vi "MU Get Config.vi"(8 "error in (no error)":errorcluster, 10 "configuration":u32, 11 "handle":u64) -> (0 "error out (no error)":errorcluster, 2 "value":u32, 3 "function return":u32)   [LabVIEW 2017, in "MU_3SL_interface.lvlib"]
uses:
  MU_3SL_interface.lvlib
  lib/MU_3SL_interface.dll
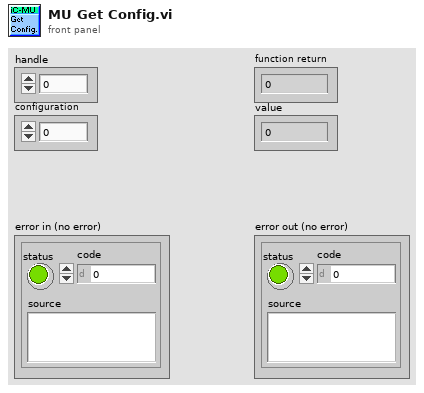
[diagram p1: front panel]
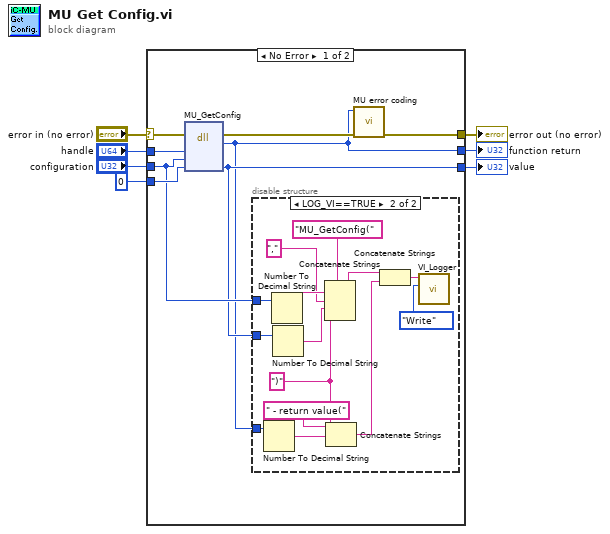
[diagram p0: block diagram]
diagram:
  n1 = case shown="No Error" "error in (no error)" {
    selector: "error in (no error)" -> [w13 w31]
    tunnel: [w8 w30] -> w7
    tunnel: "handle" -> [w11 _]
    tunnel: "configuration" -> [w10 _]
    tunnel: [w9 w30] -> w4
    tunnel: [w14 w31] -> w3
    tunnel: u32 0 ("pulValue") -> [w12 w30]
    frame No Error {
      n2 = dll-call lib="C:/Users/bes/AppData/Roaming/work/mu_9so/icsubmodules/soft_mu_3sl_master/lv_interface/lib/MU_3SL_interface**.*" fn="MU_GetConfig"(error in=w13, "handle"=w11, "configuration"=w10, "value"=w12) -> (error out=w15:errorcluster, "return type"=w8:u32, "value"=w9:u32)  [unwired: 4 in, 1 out]
      n3 = disable-structure shown="LOG_VI==TRUE" {
        disable-tunnel: w8 -> [_ w27]
        disable-tunnel: w10 -> [_ w22]
        disable-tunnel: w9 -> [_ w19]
        frame condition #0 {
        }
        frame condition #1 (active) {
          w16 = ")" ("string")
          n4 = Number To Decimal String(number=w27) -> (decimal integer string=w26:string)  [unwired: 1 in]
          n5 = Number To Decimal String(number=w22) -> (decimal integer string=w21:string)  [unwired: 1 in]
          n6 = Number To Decimal String(number=w19) -> (decimal integer string=w18:string)  [unwired: 1 in]
          n7 = Concatenate Strings("MU_GetConfig(" ("Info in"), w21, "," ("string"), w18, w16) -> (w25:string)
          n8 = Concatenate Strings(" - return value(" ("string"), w26, w16) -> (w24:string)
          n9 = Concatenate Strings(w25, w24) -> (w23:string)
          n10 = call "VI_Logger.vi"("Action (Read)"=enum16{"Write", "Read"}."Write", "Info in"=w23) -> ()  [unwired: 8 in, 2 out]
        }
      }
      n11 = call "MU error coding.vi"("error in (no error)"=w15, "function return in"=w8) -> ("error out"=w14:errorcluster)  [unwired: 9 in]
    }
    frame Error {
    }
  }
  "function return" <- w7
  "value" <- w4
  "error out (no error)" <- w3
